vi "PB_Cburn_Spectrum.vi"(0 "Spectrum Parameters":T1={"Window 1 time (s)"=0.012, "Window 2 time (s)"=5e-06, "Window 3 time (s) "=0.02, "Window 4 time (s)"=5e-07, "Path to SpectrumBurn"=path "C:/Users/Loncar/Desktop/ESR VIs - Srujan/Sam Kim/PB/ESRFreq.exe", "Window 5 time (s)"=1e-07, "Window 6 time (s)"=5e-08, "Window 1 active channels"=[FALSE, TRUE], "Window 2 active channels"=[], "Window 3 active channels "=[FALSE, FALSE, TRUE], "Window 4 active channels"=[TRUE, FALSE, TRUE], "Window 5 active channels"=[FALSE, FALSE, TRUE], "Window 6 active channels"=[]}, 1 "# scans before track":i32=50) -> (7 "String":string)   [LabVIEW 2012]
uses:
  Spectrum Window Parameters.ctl
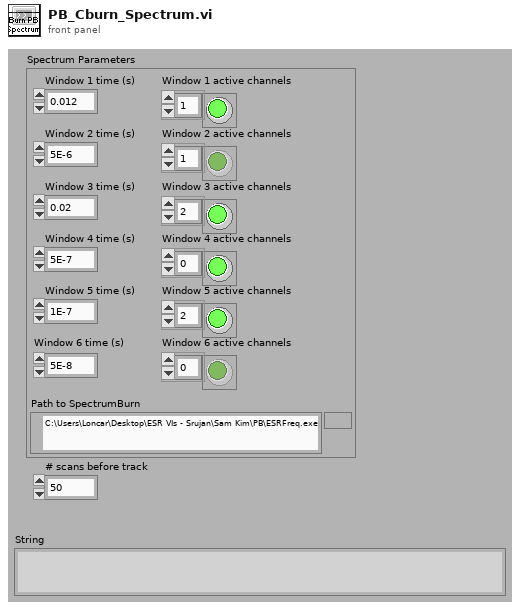
[diagram p1: front panel]
types:
  T1 = typedef "Spectrum Window Parameters.ctl" = cluster{"Window 1 time (s)":dbl, "Window 2 time (s)":dbl, "Window 3 time (s) ":dbl, "Window 4 time (s)":dbl, "Path to SpectrumBurn":path, "Window 5 time (s)":dbl, "Window 6 time (s)":dbl, "Window 1 active channels":bool[], "Window 2 active channels":bool[], "Window 3 active channels ":bool[], "Window 4 active channels":bool[], "Window 5 active channels":bool[], "Window 6 active channels":bool[]}
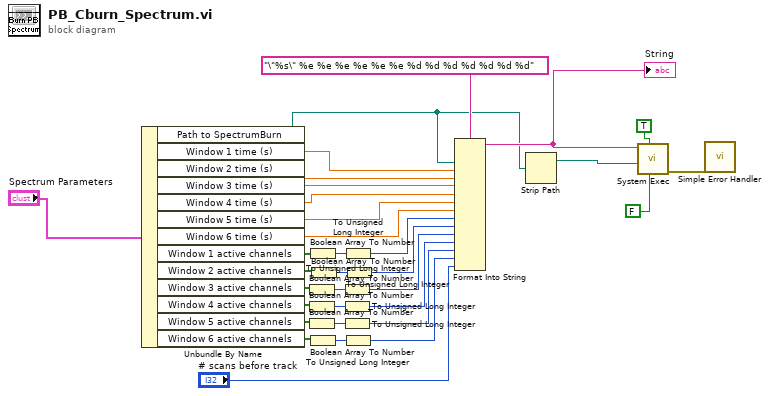
[diagram p0: block diagram]
diagram:
  n1 = Unbundle By Name("Spectrum Parameters") -> ("Path to SpectrumBurn"=w21:path, "Window 1 time (s)"=w24:dbl, "Window 2 time (s)"=w23:dbl, "Window 3 time (s)"=w22:dbl, "Window 4 time (s)"=w19:dbl, "Window 5 time (s)"=w18:dbl, "Window 6 time (s)"=w17:dbl, "Window 1 active channels"=w15:bool[], "Window 2 active channels"=w13:bool[], "Window 3 active channels"=w12:bool[], "Window 4 active channels"=w10:bool[], "Window 5 active channels"=w7:bool[], "Window 6 active channels"=w3:bool[])
  n2 = Boolean Array To Number(Boolean array=w12) -> (number=w30:u32)
  n3 = Boolean Array To Number(Boolean array=w10) -> (number=w9:u32)
  n4 = Boolean Array To Number(Boolean array=w7) -> (number=w6:u32)
  n5 = Boolean Array To Number(Boolean array=w15) -> (number=w16:u32)
  n6 = Boolean Array To Number(Boolean array=w3) -> (number=w4:u32)
  n7 = Boolean Array To Number(Boolean array=w13) -> (number=w29:u32)
  n8 = To Unsigned Long Integer(number=w30) -> (unsigned 32bit integer=w11:u32)
  n9 = To Unsigned Long Integer(number=w9) -> (unsigned 32bit integer=w8:u32)
  n10 = To Unsigned Long Integer(number=w6) -> (unsigned 32bit integer=w5:u32)
  n11 = To Unsigned Long Integer(number=w16) -> (unsigned 32bit integer=w14:u32)
  n12 = To Unsigned Long Integer(number=w4) -> (unsigned 32bit integer=w2:u32)
  n13 = To Unsigned Long Integer(number=w29) -> (unsigned 32bit integer=w28:u32)
  n14 = Format Into String(format string="\"%s\" %e %e %e %e %e %e %d %d %d %d %d %d %d", w21, w24, w23, w22, w19, w18, w17, w14, w28, w11, w8, w5, w2, "# scans before track") -> (resulting string=w26:string)  [unwired: 2 in, 1 out]
  "String" <- w26
  n15 = Strip Path(path=w21) -> (stripped path=w33:path)  [unwired: 1 out]
  n16 = call <vilib>:"System Exec.vi"("run minimized? (F)"=FALSE ("Wait until done"), "wait until completion? (T)"=TRUE ("Wait until done"), "working directory"=w33, "command line"=w26) -> ("error out"=w25:errorcluster)  [unwired: 4 in, 3 out]
  n17 = call <vilib>:"Simple Error Handler.vi"("error in (no error)"=w25) -> ()  [unwired: 4 in, 5 out]
